vi "Processed_Bytes_To_ES_Packet.vi"(3 "error in (no error)":errorcluster, 4 "Processed_Bytes":u8[](array[numeric]), 5 "ES Packet In":T2) -> (0 "error out":errorcluster, 1 "ES Param Out":T1, 2 "ES Packet Out":T2)   [LabVIEW 2017]
uses:
  Controls/Packet/Packet.ctl
  Controls/Packet/Packet_Direction.ctl
  Controls/Packet/Packet_Type.ctl
  Controls/Packet/Packet_Priority.ctl
  Controls/Control Packets/ES_Param.ctl
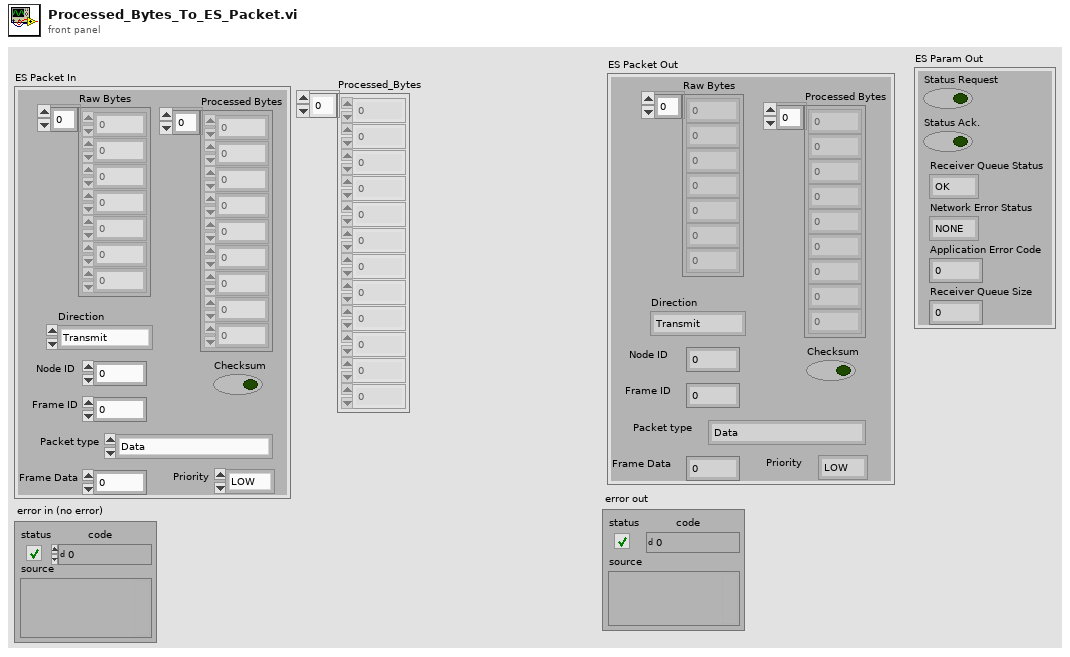
[diagram p1: front panel]
types:
  T1 = typedef "ES_Param.ctl" = cluster{"Status Request":bool, "Status Ack.":bool, "Receiver Queue Status":enum16{"OK", "EMPTY", "FULL"}, "Network Error Status":enum16{"NONE", "CONNECTION_ALREADY_OPEN", "CONNECTION_ALREADY_CLOSED", "INVALID_FRAME_REQUEST"}, "Application Error Code":u16, "Receiver Queue Size":i32}
  T2 = typedef "Packet.ctl" = cluster{"Raw Bytes":u8[], "Checksum":bool, "Direction":T3, "Processed Bytes":u8[], "Node ID":u8, "Packet type":T4, "Frame Data":u32, "Priority":T5, "Frame ID":u8}
  T3 = typedef "Packet_Direction.ctl" = enum16{"Transmit", "Receive", "Bidirectional"}
  T4 = typedef "Packet_Type.ctl" = enum16{"Data", "Connection Management", "Remote Request", "Error/Status"}
  T5 = typedef "Packet_Priority.ctl" = enum16{"LOW", "HIGH"}
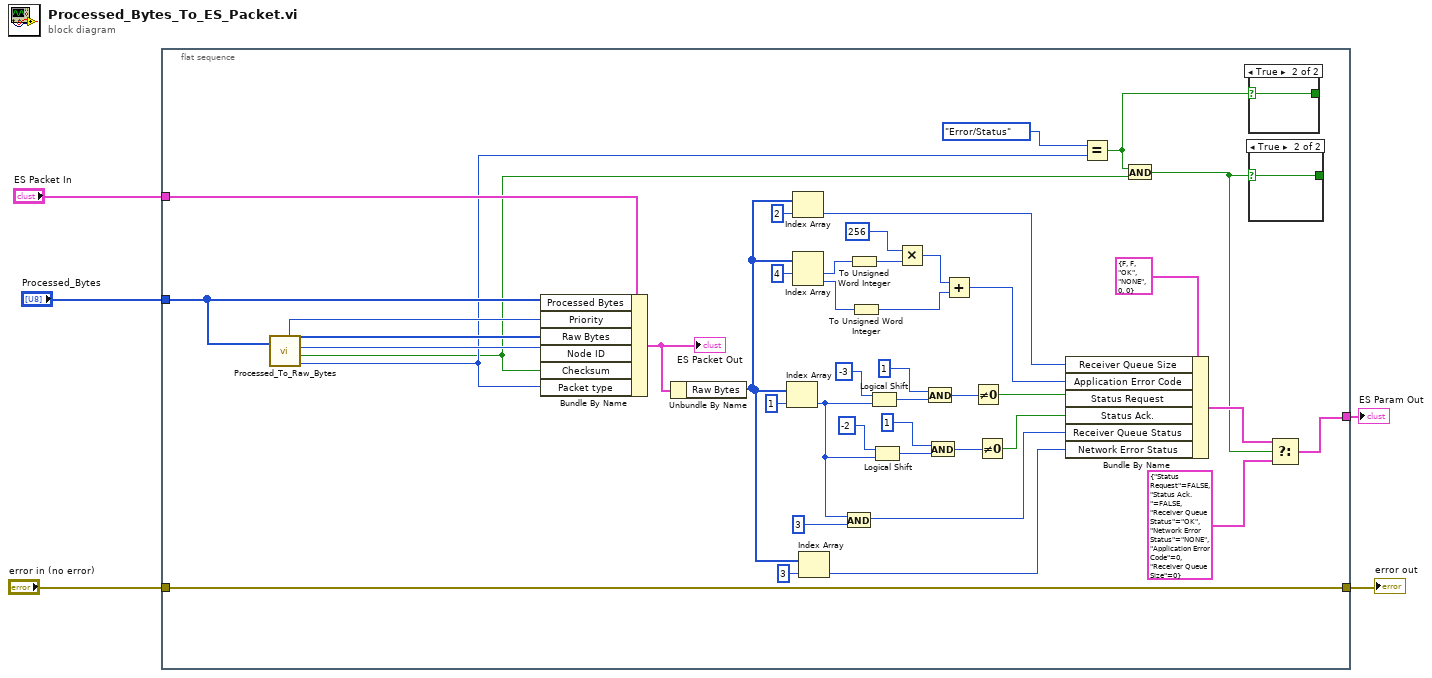
[diagram p0: block diagram]
diagram:
  n1 = flat-sequence {
    tunnel: "error in (no error)" -> [w42]
    tunnel: "ES Packet In" -> [w48]
    tunnel: "Processed_Bytes" -> [w47]
    tunnel: [w42] -> w1
    tunnel: [w8] -> w2
    frame #0 {
      n2 = call "Processed_To_Raw_Bytes.vi"("Processed Bytes"=w47) -> ("Packet Type"=w13:T4, "Checksum"=w11:bool, "Node ID"=w44:u8, "Raw Bytes"=w45:u8[], "Priority"=w46:T5)  [unwired: 1 in]
      n3 = Bundle By Name(cluster=w48, "Processed Bytes"=w47, "Priority"=w46, "Raw Bytes"=w45, "Node ID"=w44, "Checksum"=w11, "Packet type"=w13) -> (w43:T2)
      "ES Packet Out" <- w43
      n4 = Unbundle By Name(w43) -> ("Raw Bytes"=w18:u8[])
      n5 = Index Array(array=w18, index=1) -> (element=w34:u8)
      n6 = Index Array(array=w18, index=2) -> (element=w16:u8)
      n7 = Index Array(array=w18, index #1=4 ("index")) -> (element #1=w26:u8, element #2=w25:u8)  [unwired: 1 in]
      n8 = Index Array(array=w18, index=3) -> (element=w14:u8)
      n9 = And(x=w34, y=u8 3) -> (x .and. y?=w15:u8)
      n10 = To Unsigned Word Integer(number=w26) -> (unsigned 16bit integer=w24:u16)
      n11 = To Unsigned Word Integer(number=w25) -> (unsigned 16bit integer=w21:u16)
      n12 = Logical Shift(y=i16 -3, x=w34) -> (x << y=w39:u8)
      n13 = Logical Shift(y=i16 -2, x=w34) -> (x << y=w36:u8)
      n14 = Multiply(x=u16 256, y=w24) -> (x*y=w22:u16)
      n15 = And(x=u8 1, y=w39) -> (x .and. y?=w32:u8)
      n16 = And(x=u8 1, y=w36) -> (x .and. y?=w31:u8)
      n17 = Add(x=w22, y=w21) -> (x+y=w20:u16)
      n18 = Not Equal To 0?(x=w32) -> (x != 0?=w30:bool)
      n19 = Not Equal To 0?(x=w31) -> (x != 0?=w29:bool)
      n20 = Bundle By Name(cluster=T1 {"Status Request"=FALSE, "Status Ack."=FALSE, "Receiver Queue Status"=enum."OK", "Network Error Status"=enum."NONE", "Application Error Code"=0, "Receiver Queue Size"=0} ("Cluster"), "Receiver Queue Size"=w16, "Application Error Code"=w20, "Status Request"=w30, "Status Ack."=w29, "Receiver Queue Status"=w15, "Network Error Status"=w14) -> (w9:T1)
      n21 = Equal?(x=Packet_Type."Error/Status", y=w13) -> (x = y?=w6:bool)
      n22 = And(x=w6, y=w11) -> (x .and. y?=w7:bool)
      n23 = case shown="True" w6 {
        selector: w6 -> [w49 w50]
        tunnel: [w49 w50] -> _
        frame False {
        }
        frame True {
        }
      }
      n24 = case shown="True" w7 {
        selector: w7 -> [w51 w52]
        tunnel: [w51 w52] -> _
        frame False {
        }
        frame True {
        }
      }
      n25 = Select(t=w9, s=w7, f=T1 {"Status Request"=FALSE, "Status Ack."=FALSE, "Receiver Queue Status"=enum."OK", "Network Error Status"=enum."NONE", "Application Error Code"=0, "Receiver Queue Size"=0}) -> (s? t:f=w8:T1)
    }
  }
  "ES Param Out" <- w2
  "error out" <- w1
